vi "helper-collect-icc-sensors.vi"(6 "Update Virtual? (T)":bool=TRUE, 7 "Caller":string="OCS_CHECK", 8 "error in":errorcluster, 9 "path format (ie. OCS\\\\DB\\\\%s.*)":string, 10 "Section (IOnode prefix)":string, 11 "IOnodes (AI)":string[](array[string])) -> (0 "error out":errorcluster, 2 "results numeric":dbl[](array[numeric]), 3 "results report":string[](array[string]))   [LabVIEW 2024]
uses:
  io.interface.serial.vi
  Polymorphics/variantCtrlIo.vi
  globals/globals-engine.vi
  util.environment.vi
  util-address-parser.vi
  util-address-builder.vi
  util.DO.ToString.vi
  Polymorphics/io.command-builder.vi
  Polymorphics/io.command-builder.DO.vi
  Polymorphics/io.command-builder.AI.vi
  Polymorphics/io.command-builder.DI.vi
  io.frame.vi
  io.visa.vi
  io.responseValidator.vi
  Polymorphics/io.command-parser.DI.vi
  Polymorphics/io.command-parser.AI.vi
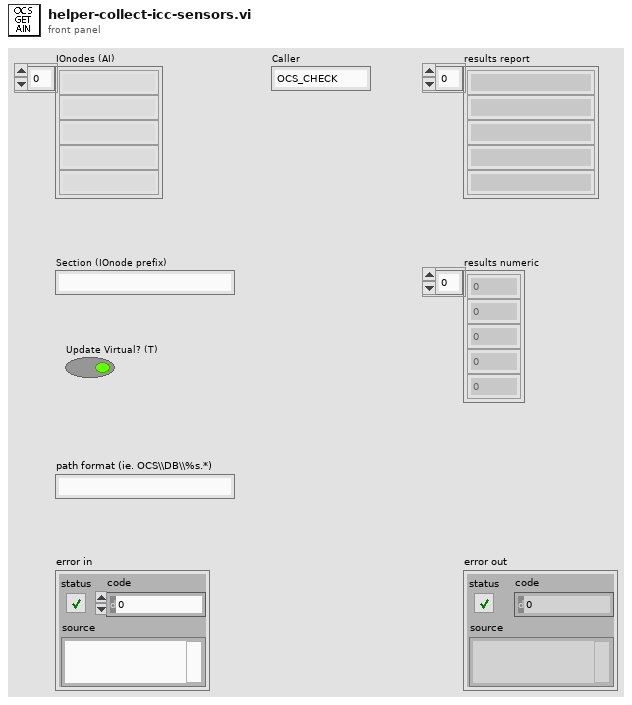
[diagram p1: front panel]
types:
  T1 = typedef "IONode.ctl" = cluster{"ADDR":T2, "Label":string, "Type":T3, "Mode":T4, "Value":string, "Tags":string, "calibration":T5[]}
  T2 = typedef "type.address.ctl" = u16
  T3 = typedef "enum.io.type.ctl" = enum16{"Type", "DI", "DO", "AI", "AO", "VL", "BUF"}
  T4 = typedef "enum.io.mode.ctl" = enum16{"Mode", "RIO", "SIM"}
  T5 = typedef "typeXyPoint.ctl" = cluster{"X":dbl, "Y":dbl}
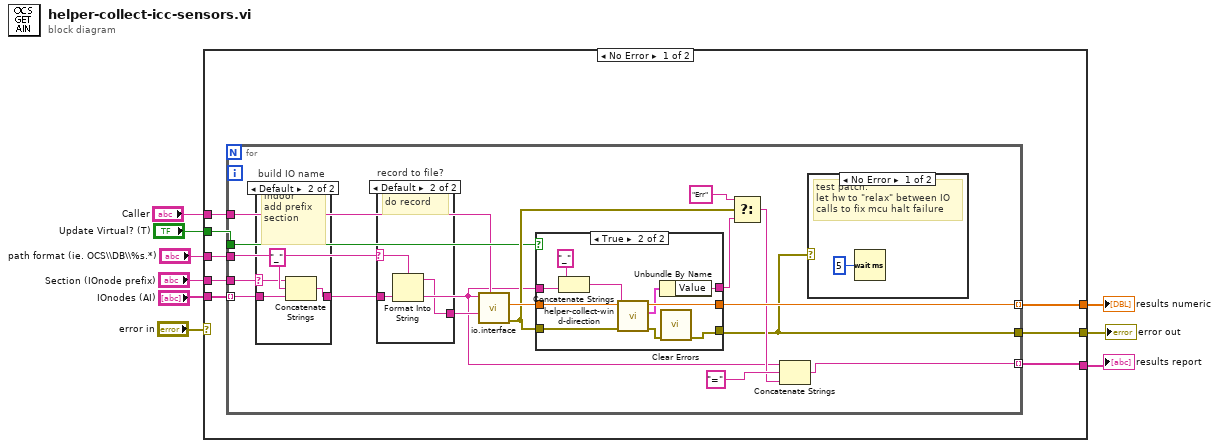
[diagram p0: block diagram]
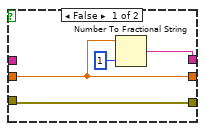
[diagram p4: hidden frame]
diagram:
  n1 = case shown="No Error" "error in" {
    selector: "error in" -> [_ w57]
    tunnel: [w17 w57] -> w9
    tunnel: [w16 _] -> w8
    tunnel: "IOnodes (AI)" -> [w15 _]
    tunnel: "Section (IOnode prefix)" -> [w14 _]
    tunnel: "path format (ie. OCS\\\\DB\\\\%s.*)" -> [w13 _]
    tunnel: [w12 _] -> w3
    tunnel: "Update Virtual? (T)" -> [w11 _]
    tunnel: "Caller" -> [w10 _]
    frame No Error {
      n2 = for {
        tunnel: w15 -> [w31] mode=indexing
        tunnel: [w20] -> w17
        tunnel: [w32] -> w12 mode=indexing
        tunnel: [w29] -> w16 mode=indexing
        tunnel: w14 -> [w24]
        tunnel: w13 -> [w21]
        tunnel: w11 -> [w22]
        tunnel: w10 -> [w19]
        n3 = case "build IO name" shown="Default" w24 {
          selector: w24 -> [_ w53]
          tunnel: w31 -> [w52 w56]
          tunnel: [w52 w55] -> w18
          frame "" {
            # "outdoor"
          }
          frame Default {
            # "indoor\nadd prefix\nsection"
            n4 = Concatenate Strings(w53, "_" ("string"), w56) -> (w55:string)
          }
        }
        n5 = case "record to file?" shown="Default" w21 {
          selector: w21 -> [_ w35]
          tunnel: w18 -> [_ w37]
          tunnel: [_ w36] -> w23
          frame "" {
            # "skip record to file"
          }
          frame Default {
            # "do record"
            n6 = Format Into String(format string=w35, w37) -> (resulting string=w36:string)  [unwired: 2 in, 1 out]
          }
        }
        n7 = call "io.interface.vi"("Caller"=w19, "record filename.* (disabled if empty)"=w23, "IO Name in"=w18) -> ("error out"=w28:errorcluster, "Value out"=w33:dbl)  [unwired: 3 in, 4 out]
        n8 = case shown="True" w22 {
          tunnel: w33 -> [w39 w51]
          tunnel: [w39 w50] -> w32
          tunnel: w28 -> [w41 w48]
          tunnel: [w38 w47] -> w27
          tunnel: [w41 w45] -> w20
          tunnel: w18 -> [_ w43]
          frame False {
            n9 = Number To Fractional String(number=w39, precision (6)=i16 1) -> (F-format string=w38:string)  [unwired: 2 in]
          }
          frame True {
            n10 = Concatenate Strings("_" ("string"), w43) -> (w44:string)
            n11 = call "helper-collect-wind-direction.vi"("error in"=w48, "Result Virtual Name"=w44, "Value in"=w51) -> ("error out"=w46:errorcluster, "Result Node"=w49:T1, "Result"=w50:dbl)  [unwired: 5 in, 1 out]
            n12 = Unbundle By Name(w49) -> ("Value"=w47:string)
            n13 = call <vilib>:"Clear Errors.vi"("error in (no error)"=w46) -> ("error out"=w45:errorcluster)  [unwired: 5 in, 1 out]
          }
        }
        n14 = Select(t="Err", s=w28, f=w27) -> (s? t:f=w26:string)
        n15 = Concatenate Strings(w18, "=" ("string"), w26) -> (w29:string)
        n16 = case shown="No Error" w20 {
          frame No Error {
            # "test patch:\nlet hw to \"relax\" between IO calls to fix mcu halt failure"
            n17 = Wait (ms)(milliseconds to wait=u32 5) -> ()  [unwired: 1 out]
          }
          frame Error {
          }
        }
      }
    }
    frame Error {
    }
  }
  "error out" <- w9
  "results report" <- w8
  "results numeric" <- w3
